vi "ini_sesion.vi"(8 "error in (no error)":errorcluster, 11 "5785_3.2GHz_one channel in":refnum<class "5785_3.2GHz_one channel.lvclass">) -> (0 "error out":errorcluster, 3 "5785_3.2GHz_one channel out":refnum<class "5785_3.2GHz_one channel.lvclass">)   [LabVIEW 2021, in "5785_3.2GHz_one channel.lvclass"]
uses:
  5785_3.2GHz_one channel.lvclass
  5785_3.2GHz_one channel.lvclass/5785_3.2GHz_one channel.ctl
  <instrlib>/FlexRIO/API/Host/v1/NI FlexRIO/API/Reference Clock Source.ctl
  <vilib>/FPGAPlugInAG/PXIe-5785 (KU060)/niLvFpga_Open_PXIe-5785 (KU060).vi
  <vilib>/rvi/interface/common/dynamic/niFpgaDynamicAddResources.vi
  <instrlib>/FlexRIO/API/Host/v1/NI FlexRIO/API/Configure Reference Clock.vi
  <vilib>/Utility/error.llb/Error Cluster From Error Code.vi
  <vilib>/rvi/errors/niLvFpgaAdjustHostInterfaceError.vi
  <instrlib>/FlexRIO/API/Host/v1/NI FlexRIO/API/Get Property Reference - Fpga Small.vi
  <vilib>/rvi/interface/common/niFpgaWaitOnOcc.vi
  <vilib>/rvi/interface/nirviOpenFPGA/nirviOpenFPGA.xnode
  FPGA Bitfiles/5785_3200MHz_multi emitter 8 and 4.lvbitx
  FPGA Bitfiles/5785_Multi_Emitter_3GHz_IBW.lvbitx
  <vilib>/rvi/interface/nirviReadWriteControl/nirviReadWriteControl.xnode
  <vilib>/rvi/interface/nirviMethod/nirviMethod.xnode
  <instrlib>/FlexRIO/API/Host/v1/NI FlexRIO API v1.lvlib
  <resource>/objmgr/niflexrioapiStream.rc
  <resource>/objmgr/niflexrioapi.rc
  <vilib>/rvi/errors/niLvFpgaMergeErrorWithErrorCode.vi
  <resource>/objmgr/niflexrioapiChannel.rc
  <vilib>/FPGAPlugInAG/Dynamic/niLvFpga_StopFifo_Dynamic.vi
  <vilib>/FPGAPlugInAG/Dynamic/niLvFpga_ConfigureFifo_Dynamic.vi
  NiFpgaLv.dll
  <vilib>/rvi/interface/Simulation/niFpgaSimulationCallBeginRW.vi
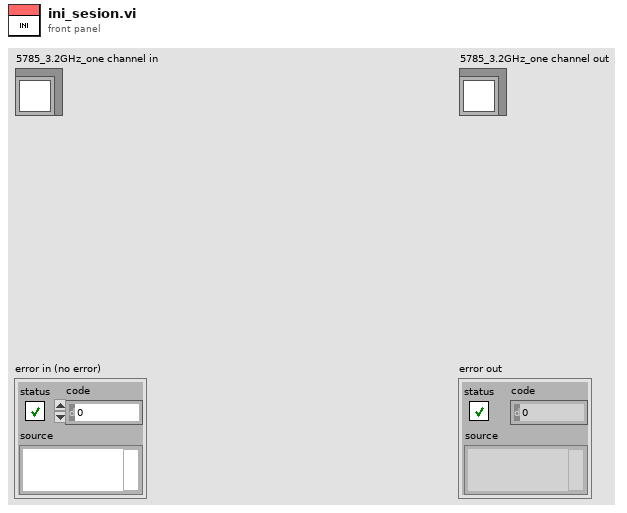
[diagram p1: front panel]
types:
  T1 = typedef "nirio_resource_hc.ctl" = tag
  T2 = typedef "NI FlexRIO API v1.lvlib/Reference Clock Source.ctl" = i32
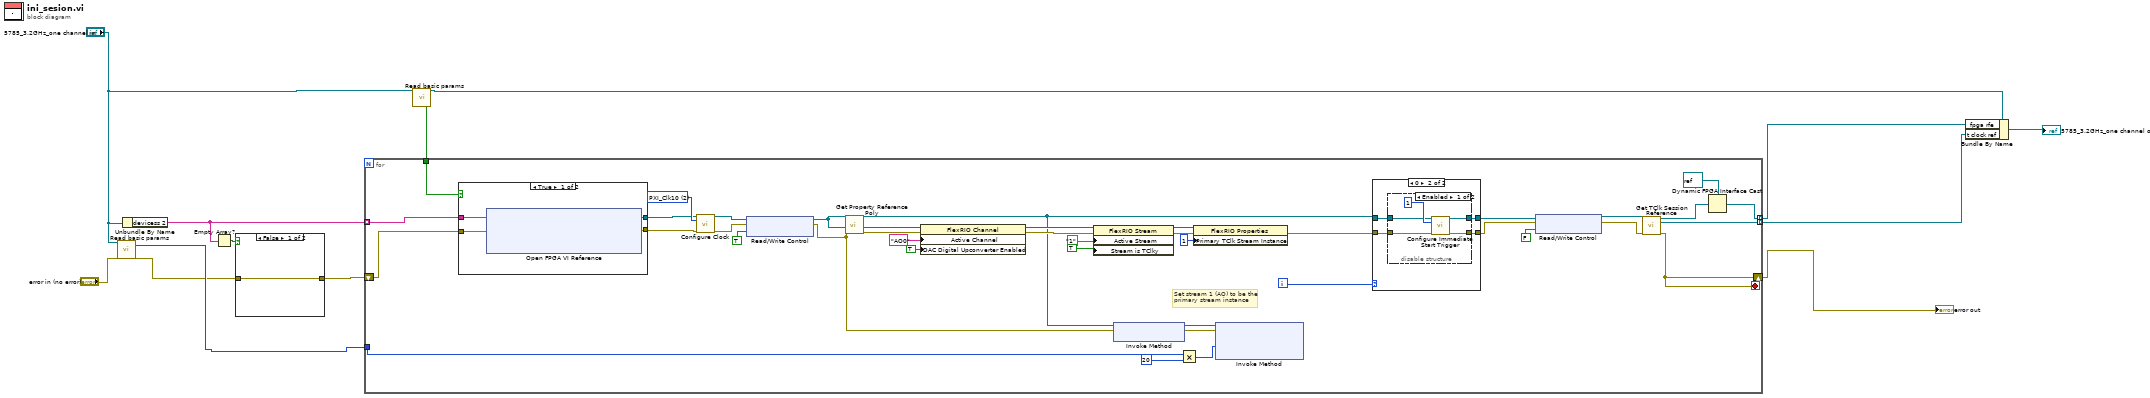
[diagram p0: block diagram]
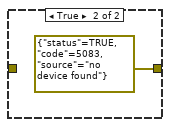
[diagram p2: hidden frame]
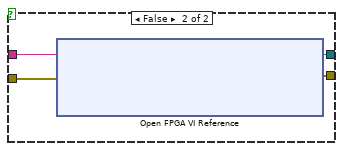
[diagram p3: hidden frame]
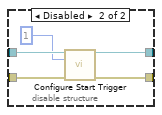
[diagram p5: hidden frame]
diagram:
  n1 = call-dynamic "Read basic params.vi"("device_type in"="5785_3.2GHz_one channel in", "error in (no error)"="error in (no error)") -> ("buffer size"=w7:u32, "error out"=w5:errorcluster)  [unwired: 11 in, 5 out]
  n2 = Unbundle By Name("5785_3.2GHz_one channel in") -> ("devicess 2"=w12:T1[])
  n3 = Empty Array?(array=w12) -> (empty?=w11:bool)
  n4 = case shown="False" w11 {
    tunnel: [w14 errorcluster {"status"=TRUE, "code"=5083, "source"="no device found"} ("error in (no error)")] -> w10
    tunnel: w5 -> [w14 _]
    frame False {
    }
    frame True {
    }
  }
  n5 = call-dynamic "Read basic params.vi"("device_type in"="5785_3.2GHz_one channel in") -> ("use arb files"=w2:bool, "device_type out"=w3:refnum<class "5785_3.2GHz_one channel.lvclass">)  [unwired: 12 in, 5 out]
  n6 = for {
    tunnel: [w21] -> w1 mode=indexing
    shift-right: [w33] -> w9
    shift-left: w10 -> [w46]
    tunnel: [w49] -> w13 mode=indexing
    tunnel: w7 -> [w45]
    tunnel: w12 -> [w37] mode=indexing
    tunnel: w2 -> [w24]
    i -> [w47]
    stop <- w33 stop-if-true
    w36 = T2 2 items=["Default", "Onboard", "PXI_Clk10", "External", "None", "Baseboard Reference"] ("reference clock source")
    # "Set stream 1 (AO) to be the\nprimary stream instance"
    n7 = case shown="True" w24 {
      tunnel: w46 -> [w58 w62]
      tunnel: w37 -> [w57 w61]
      tunnel: [w56 w60] -> w35
      tunnel: [w55 w59] -> w34
      frame True {
        n8 = xnode "Open FPGA VI Reference"("error in"=w58, "resource name"=w57) -> ("FPGA VI Reference Out"=w56:refnum<k20>, "error out"=w55:errorcluster)
      }
      frame False {
        n9 = xnode "Open FPGA VI Reference"("error in"=w62, "resource name"=w61) -> ("FPGA VI Reference Out"=w60:refnum<k20>, "error out"=w59:errorcluster)
      }
    }
    n10 = call-poly <instrlib>:"Configure Clock.vi"("fpga interface in"=w35, "reference clock source"=w36, "error in"=w34) -> ("fpga interface out"=w19:refnum<k20>, "error out"=w18:errorcluster)  [unwired: 11 in]
    n11 = xnode "Read/Write Control"("FPGA VI Reference In"=w19, "error in"=w18, "reset system clock"=TRUE) -> ("FPGA VI Reference Out"=w16:refnum<k20>, "error out"=w17:errorcluster)
    n12 = call-poly <instrlib>:"Get Property Reference Poly.vi"("error in (no error)"=w17, "fpga interface in"=w16) -> ("error out"=w40:errorcluster, "property reference"=w41:refnum<k20>)  [unwired: 4 in, 1 out]
    n13 = property class="FlexRIO Channel"(reference=w41, error in=w40, "Active Channel"="AO0", "DAC Digital Upconverter Enabled"=TRUE ("Analog Output:DAC Digital Upconverter Enabled")) -> (reference out=w39:refnum<k20>, error out=w38:errorcluster)
    n14 = property class="FlexRIO Stream"(reference=w39, error in=w38, "Active Stream"="1", "Stream is TClky"=TRUE ("Configuration:Stream is TClky")) -> (reference out=w52:refnum<k20>, error out=w51:errorcluster)
    n15 = xnode "Invoke Method"("FPGA VI Reference In"=w16, "error in"=w17) -> ("FPGA VI Reference Out"=w26:refnum<k20>, "error out"=w27:errorcluster)
    n16 = Multiply(x=w45, y=u32 20) -> (x*y=w44:u32)
    n17 = property class="FlexRIO Properties"(reference=w52, error in=w51, "Primary TClk Stream Instance"=1 ("Device:Primary TClk Stream Instance")) -> (error out=w48:errorcluster)  [unwired: 1 out]
    n18 = xnode "Invoke Method"("FPGA VI Reference In"=w26, "error in"=w27, "Requested Depth"=w44) -> ()  [unwired: 3 out]
    n19 = case shown="0" w47 {
      tunnel: w16 -> [w64 w68]
      tunnel: [w64 w67] -> w32
      tunnel: [w63 w66] -> w29
      tunnel: w48 -> [w63 w65]
      frame 1, Default {
      }
      frame 0 {
        n20 = disable-structure shown="Enabled" {
          disable-tunnel: w68 -> [w72 w78]
          disable-tunnel: [w71 w76] -> w67
          disable-tunnel: [w70 w75] -> w66
          disable-tunnel: w65 -> [w69 w74]
          frame Enabled {
            n21 = call <instrlib>:"Configure Immediate Start Trigger.vi"("fpga interface in"=w72, "trigger instance"=u32 1, "error in"=w69) -> ("fpga interface out"=w71:refnum<k20>, "error out"=w70:errorcluster)  [unwired: 10 in, 1 out]
          }
          frame Disabled {
            n22 = call-poly <instrlib>:"Configure Start Trigger.vi"("fpga interface in"=w78, "trigger instance"=u32 1, "error in"=w74) -> ("fpga interface out"=w76:refnum<k20>, "error out"=w75:errorcluster)  [unwired: 10 in, 1 out]
          }
        }
      }
    }
    n23 = xnode "Read/Write Control"("FPGA VI Reference In"=w32, "error in"=w29, "reset system clock"=FALSE) -> ("FPGA VI Reference Out"=w31:refnum<k20>, "error out"=w30:errorcluster)
    n24 = call <instrlib>:"Get TClk Session Reference.vi"("fpga interface in"=w31, "error in"=w30) -> ("fpga interface out"=w22:refnum<k20>, "tclk session reference"=w49:refnum<k20>, "error out"=w33:errorcluster)  [unwired: 11 in]
    n25 = Dynamic FPGA Interface Cast(Session In=refnum<k20> refnum ("FPGA VI Reference Out"), Type=w22) -> (Session Out=w21:refnum<k20>)
  }
  "error out" <- w9
  n26 = Bundle By Name(cluster=w3, "fpga rfe"=w1, "t clock ref"=w13) -> (→"5785_3.2GHz_one channel out":refnum<class "5785_3.2GHz_one channel.lvclass">)
